vi "Pos_iniciales1.vi"() -> ()   [LabVIEW 2020]
panel:
  in  "Pos_Iniciales1":T1
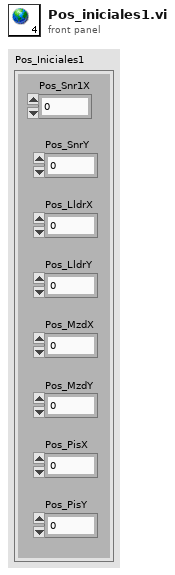
[diagram p1: front panel]
types:
  T1 = cluster{"Pos_Snr1X":dbl, "Pos_SnrY":dbl, "Pos_LldrX":dbl, "Pos_LldrY":dbl, "Pos_MzdX":dbl, "Pos_MzdY":dbl, "Pos_PisX":dbl, "Pos_PisY":dbl}
diagram:
